vi "FM Modulation Demo (Single tone) - Second.vi"() -> ()   [LabVIEW 2013]
uses:
  <vilib>/express/express analysis/Spectral/Block/exnSpectralBlock spectral measurements power poly.vi
  <vilib>/express/express analysis/Spectral/Block/exnSpectralBlock spectral measurements power DDT.vi
  <vilib>/express/express analysis/Spectral/XNode/ExpressSpectralMeasurementsBlockNode.xnode
panel:
  in  "WAV Sample Rate":dbl=44100.0 caption="dt"
  in  "Mod. Freq.":dbl=2000.0 caption="Frequency"
  in  "LPF Cut-Off":dbl=10000.0 caption="Lower Cut-Off"
  in  "AWGN (dB)":dbl(slide)=0.6 caption="Standard deviation" scale=-20.0..30.0
  out "Comparision":dynamicdata(graph)
  out "Baseband":dynamicdata(graph)
  out "FM FFT":dynamicdata(graph)
  out "FM Wave":dynamicdata(graph)
  in  "DC Offset":dbl=1.0
  in  "Carrier Amp.":dbl=1.0 caption="Amplitude"
  in  "stop":bool
  in  "Frequency Deviation":dbl(slide)=1.0 scale=0.0..5.0
  in  "Carrier Freq.":dbl=100000.0 caption="Frequency"
  out "After Rectifier":cluster{"f0":dbl, "df":dbl, "magnitude":dbl[]}(graph)
  # "FM Modulation"
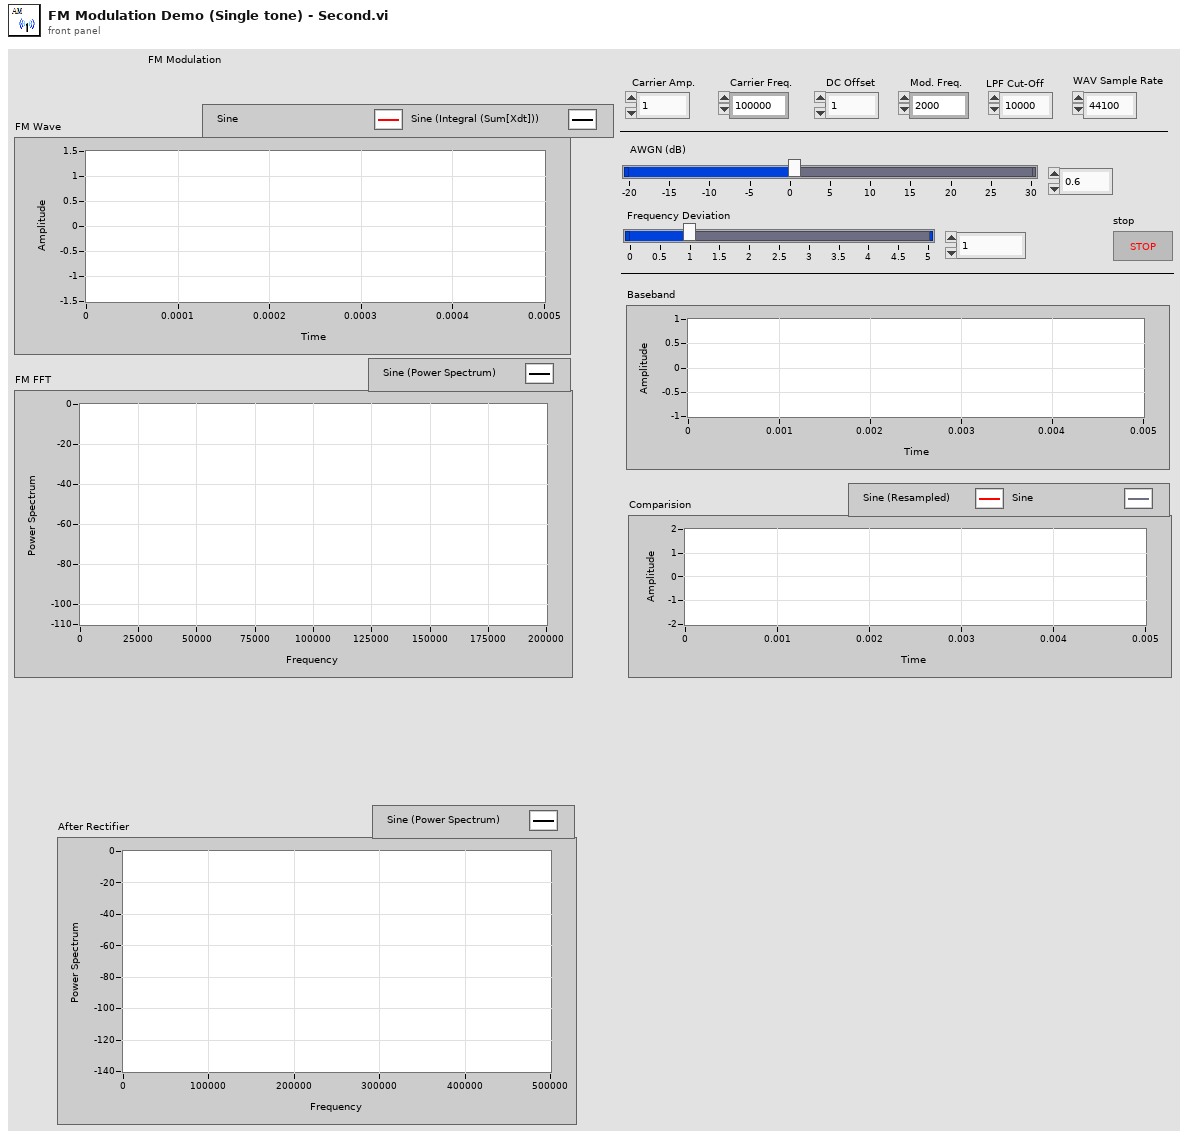
[diagram p1: front panel]
types:
  T1 = cluster{"averaging mode":u16, "weighting mode":u16, "number of averages":u32}
  T2 = cluster{"dB On (F)":bool, "unwrap phase (F)":bool, "convert to degree (F)":bool}
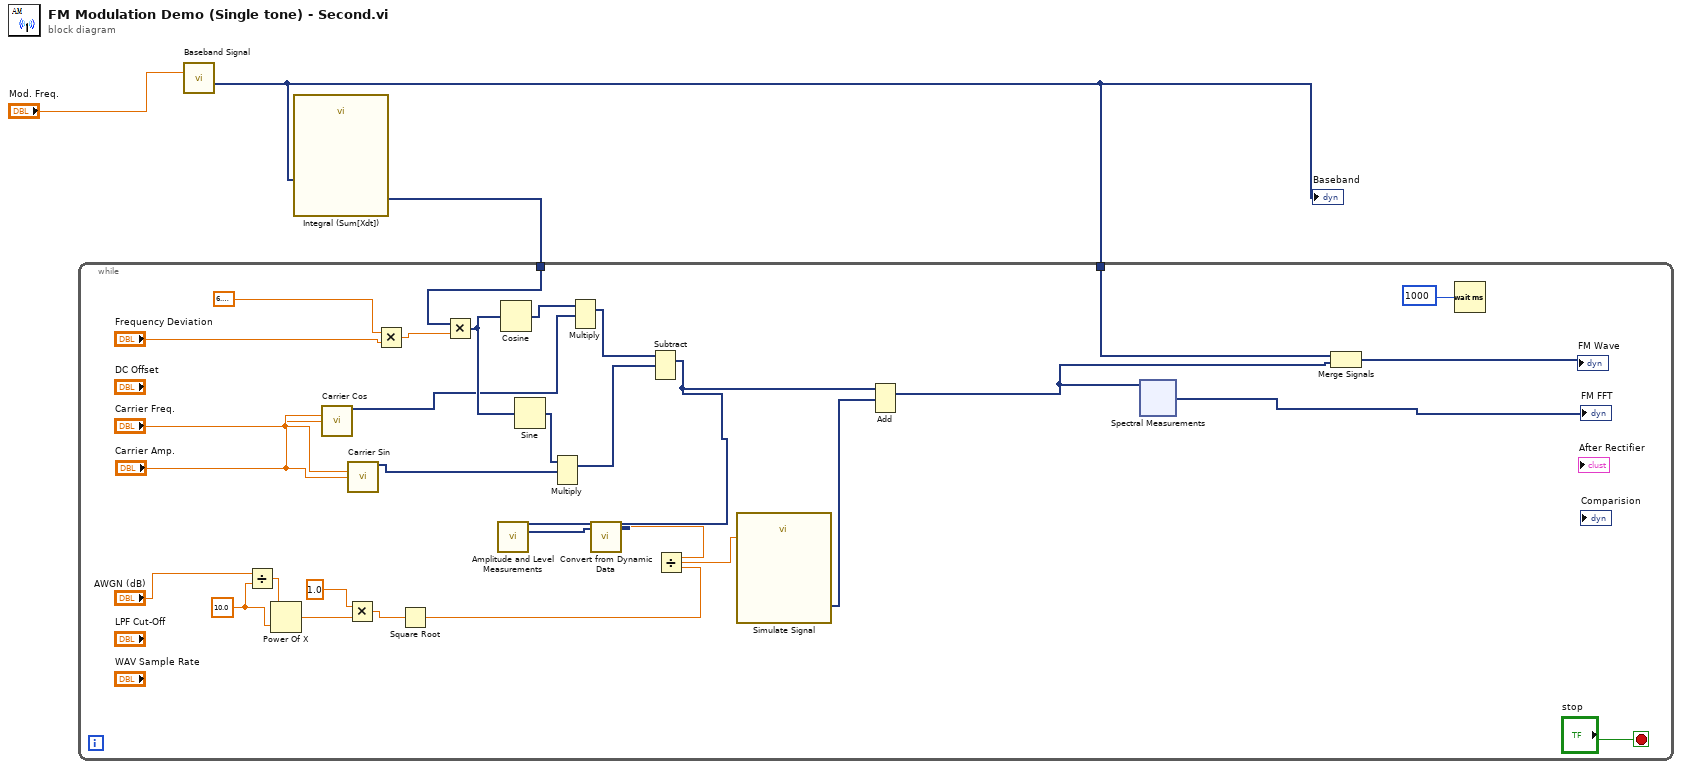
[diagram p0: block diagram]
diagram:
  n1 = call "Baseband Signal"("Frequency"="Mod. Freq.") -> ("Sine"=w2:dynamicdata)  [unwired: 13 in, 1 out]
  "Baseband" <- w2
  n2 = call "Integral (Sum[Xdt])"("Signals"=w2) -> ("Result"=w1:dynamicdata)  [unwired: 5 in, 1 out]
  n3 = while {
    tunnel: w2 -> [w11]
    tunnel: w1 -> [w15]
    stop <- "stop" stop-if-true
    w20 = 10.0
    n4 = Divide(x="AWGN (dB)", y=w20) -> (x/y=w21:dbl)
    n5 = Power Of X(1:w20, 2:w21) -> (0:w19:dbl)
    n6 = call "Carrier Cos"("Frequency"="Carrier Freq.", "Amplitude"="Carrier Amp.") -> ("Sine"=w5:dynamicdata)  [unwired: 12 in, 1 out]
    n7 = Multiply(x=1.0, y=w19) -> (x*y=w28:dbl)
    n8 = call "Carrier Sin"("Frequency"="Carrier Freq.", "Amplitude"="Carrier Amp.") -> ("Sine"=w9:dynamicdata)  [unwired: 12 in, 1 out]
    n9 = Multiply(x=6.283185307179586, y="Frequency Deviation") -> (x*y=w16:dbl)
    n10 = Square Root(x=w28) -> (sqrt(x)=w26:dbl)
    n11 = Multiply(x=w15, y=w16) -> (x*y=w8:dynamicdata)
    n12 = Cosine(x=w8) -> (cos(x)=w6:dynamicdata)
    n13 = Sine(x=w8) -> (sin(x)=w7:dynamicdata)
    n14 = Multiply(1:w9, 2:w7) -> (0:w10:dynamicdata)  [unwired: 1 in, 1 out]
    n15 = Multiply(1:w5, 2:w6) -> (0:w4:dynamicdata)  [unwired: 1 in, 1 out]
    n16 = Subtract(1:w10, 2:w4) -> (0:w12:dynamicdata)  [unwired: 1 in, 1 out]
    n17 = call "Amplitude and Level Measurements"("Signals"=w12) -> ("RMS"=w31:dynamicdata)  [unwired: 13 in, 1 out]
    n18 = call "Convert from Dynamic Data"("Dynamic Data Type"=w31) -> ("Scalar"=w27:dbl)  [unwired: 3 in]
    n19 = Divide(x=w27, y=w26) -> (x/y=w18:dbl)
    n20 = call "Simulate Signal"("Standard deviation"=w18) -> ("DC with Gaussian Noise"=w25:dynamicdata)  [unwired: 13 in, 1 out]
    n21 = Add(1:w25, 2:w12) -> (0:w24:dynamicdata)  [unwired: 1 in, 1 out]
    n22 = xnode "Spectral Measurements"("Signals"=w24) -> ("Power Spectrum"=→"FM FFT":dynamicdata)  [unwired: 1 in, 1 out]
    n23 = Merge Signals(w11, w24) -> (→"FM Wave":dynamicdata)
    n24 = Wait (ms)(milliseconds to wait=1000) -> ()  [unwired: 1 out]
  }
